vi "Align3DPointSetToPlaneArbitrary.vi"(8 "error in":errorcluster, 10 "Plane Coeffcients":T1, 11 "Point Set":T2[](array[typedef])) -> (0 "error out":errorcluster, 3 "Points Aligned to Plane":T2[](array[typedef]))   [LabVIEW 2020, in "pointset_utils.lvlib"]
uses:
  pointset_utils.lvlib
  common/Object Point (Float).ctl
  Plane Alignment Coeffecients.ctl
  Align Point Set to Plane/PlaneCoeffecients.ctl
  Align Point Set to Plane/EstimatePlaneForPointSet.vi
  Align Point Set to Plane/RotationMatrixBetweenPlanes.vi
  <vilib>/Analysis/baseanly.llb/A x Vector.vi
  <vilib>/Analysis/baseanly.llb/Mean.vi
  <vilib>/Analysis/baseanly.llb/Mean (DBL).vi
  <vilib>/Analysis/baseanly.llb/Dot Product.vi
  <vilib>/Analysis/baseanly.llb/Real Dot Product.vi
  <vilib>/Analysis/7linalg.llb/Matrix Power.vi
  <vilib>/Analysis/7linalg.llb/Real Matrix Power.vi
  <vilib>/Analysis/_algsub.llb/Matrix Norm.vi
  <vilib>/Analysis/_algsub.llb/Real Matrix Norm.vi
  <vilib>/Analysis/7linalg.llb/SVD Decomposition.vi
  <vilib>/Analysis/7linalg.llb/Real SVD Decomposition.vi
  <vilib>/Analysis/7linalg.llb/Create Special Matrix.vi
  <vilib>/Analysis/7linalg.llb/Create Special Real Matrix.vi
  <vilib>/Analysis/coordinate.llb/Cross Product.vi
  <vilib>/Utility/error.llb/Error Cluster From Error Code.vi
  <vilib>/Analysis/Matrix/Numeric/Conversions/Array To Matrix - RA2.vi
  <vilib>/Analysis/Matrix/Numeric/Multiply/Multiply - RM,R.vi
  <vilib>/Analysis/Matrix/Numeric/Add/Add - RM,RM.vi
  Align Point Set to Plane/Align Point Set to Plane.lvlib
  common/common.lvlib
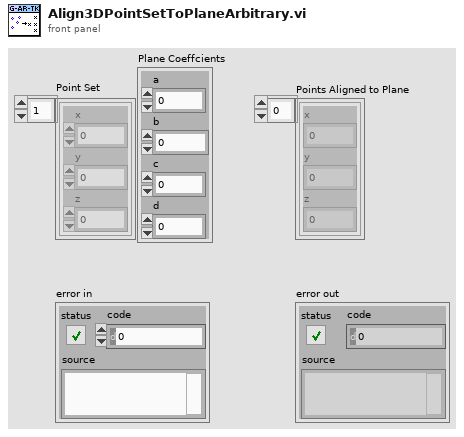
[diagram p1: front panel]
types:
  T1 = typedef "pointset_utils.lvlib/Plane Alignment Coeffecients.ctl" = cluster{"a":dbl, "b":dbl, "c":dbl, "d":dbl}
  T2 = typedef "common.lvlib/Object Point (Float).ctl" = cluster{"x":dbl, "y":dbl, "z":dbl}
  T3 = typedef "pointset_utils.lvlib/Align Point Set to Plane.lvlib/PlaneCoeffecients.ctl" = cluster{"a":dbl, "b":dbl, "c":dbl, "d":dbl}
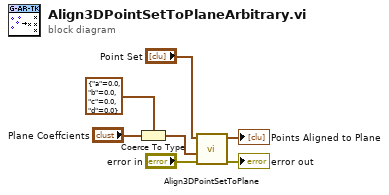
[diagram p0: block diagram]
diagram:
  n1 = Coerce To Type(0:"Plane Coeffcients", 1:T3 {"a"=0.0, "b"=0.0, "c"=0.0, "d"=0.0} ("Plane Coeffcients")) -> (2:w3:T3)
  n2 = call "Align3DPointSetToPlane.vi"("error in"="error in", "Plane Coeffcients"=w3, "Point Set"="Point Set") -> ("error out"=→"error out":errorcluster, "Points Fitted to Plane"=→"Points Aligned to Plane":T2[])  [unwired: 7 in]
